vi "iTweezers_nettest_standalone.vi"() -> ()   [LabVIEW 2010]
uses:
  iTweezers.llb/iTweezers_globals.vi
panel:
  out "IP Addresses":string[](array[string])
  out "Trap Control":bool
  out "Image Streaming":bool
  in  "stop":bool
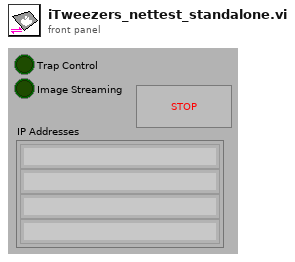
[diagram p1: front panel]
types:
  T1 = enum16{"Standard", "Buffered", "CRLF", "Immediate"}
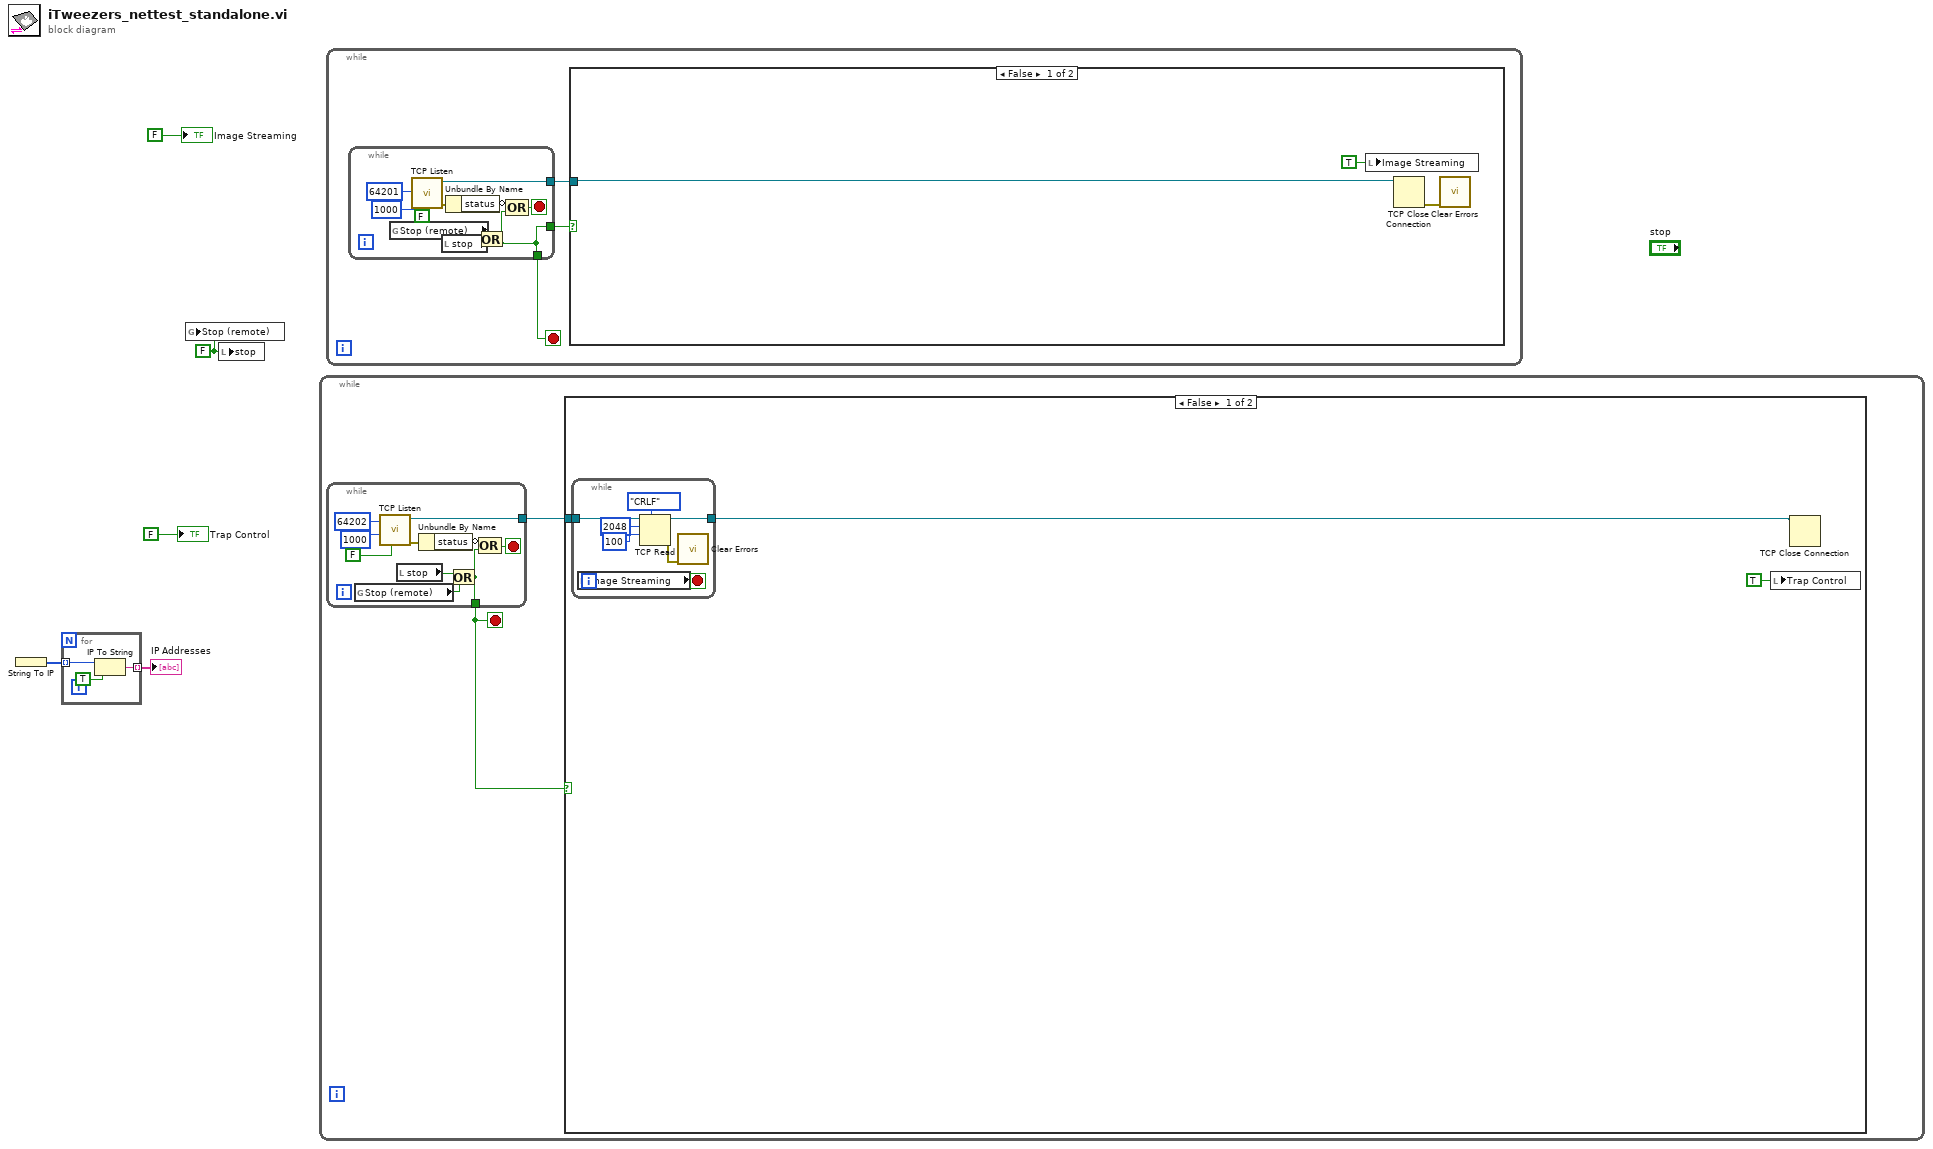
[diagram p0: block diagram]
diagram:
  w5 = FALSE ("stop")
  n1 = String To IP() -> (0:w4:u32[])  [unwired: 1 in]
  n2 = for {
    tunnel: w4 -> [w8] mode=indexing
    tunnel: [w6] -> w3 mode=indexing
    n3 = IP To String(1:TRUE ("dot notation? (F)"), 2:w8) -> (0:w6:string)
  }
  "IP Addresses" <- w3
  n4 = global write "iTweezers_globals.vi" "Stop (remote)"(w5) -> ()
  n5 = local write "stop"(w5) -> ()
  n6 = while {
    stop <- w9 stop-if-true
    n7 = while {
      tunnel: [w29] -> w10
      tunnel: [w22] -> w9
      stop <- w24 stop-if-true
      n8 = global read "iTweezers_globals.vi" "Stop (remote)"() -> (w21:bool)
      n9 = call <vilib>:"TCP Listen.vi"("resolve remote address (T)"=FALSE, "timeout ms (wait forever: -1)"=1000, "port"=u16 64202) -> ("error out"=w25:errorcluster, "connection ID"=w29:refnum<k5>)  [unwired: 2 in, 5 out]
      n10 = local read "stop"() -> (w23:bool)
      n11 = Unbundle By Name(w25) -> ("status"=w26:bool)
      n12 = Or(x=w23, y=w21) -> (x .or. y?=w22:bool)
      n13 = Compound Arithmetic op=OR(invert w26, w22) -> (w24:bool)
    }
    n14 = case shown="False" w9 {
      tunnel: w10 -> [w12 _]
      frame False {
        n15 = while {
          tunnel: [w19] -> w11
          tunnel: w12 -> [w20]
          stop <- w14 stop-if-true
          n16 = local read "Image Streaming"() -> (w14:bool)
          n17 = TCP Read(connection ID=w20, bytes to read=2048, 7:T1."CRLF" ("mode (standard)"), 9:100 ("timeout ms (25000)")) -> (connection ID out=w19:refnum<k5>, error out=w15:errorcluster)  [unwired: 1 in, 1 out]
          n18 = call <vilib>:"Clear Errors.vi"("error in (no error)"=w15) -> ()  [unwired: 6 in, 1 out]
        }
        n19 = local write "Trap Control"(TRUE ("Trap Control")) -> ()
        n20 = TCP Close Connection(connection ID=w11) -> ()  [unwired: 1 in, 3 out]
      }
      frame True {
      }
    }
  }
  n21 = while {
    stop <- w31 stop-if-true
    n22 = while {
      tunnel: [w45] -> w32
      tunnel: [w38] -> w33
      tunnel: [w38] -> w31
      stop <- w40 stop-if-true
      n23 = global read "iTweezers_globals.vi" "Stop (remote)"() -> (w37:bool)
      n24 = call <vilib>:"TCP Listen.vi"("resolve remote address (T)"=FALSE, "timeout ms (wait forever: -1)"=1000, "port"=u16 64201) -> ("error out"=w42:errorcluster, "connection ID"=w45:refnum<k5>)  [unwired: 2 in, 5 out]
      n25 = local read "stop"() -> (w39:bool)
      n26 = Unbundle By Name(w42) -> ("status"=w41:bool)
      n27 = Or(x=w37, y=w39) -> (x .or. y?=w38:bool)
      n28 = Compound Arithmetic op=OR(invert w41, w38) -> (w40:bool)
    }
    n29 = case shown="False" w33 {
      tunnel: w32 -> [w35 _]
      frame False {
        n30 = local write "Image Streaming"(TRUE ("Image Streaming")) -> ()
        n31 = TCP Close Connection(connection ID=w35) -> (error out=w36:errorcluster)  [unwired: 1 in, 2 out]
        n32 = call <vilib>:"Clear Errors.vi"("error in (no error)"=w36) -> ()  [unwired: 7 out]
      }
      frame True {
      }
    }
  }
  "Image Streaming" <- FALSE
  "Trap Control" <- FALSE
